vi "Break on Unsupported Target.vi"   [LabVIEW 2020, in "common.lvlib"]
uses:
  common.lvlib
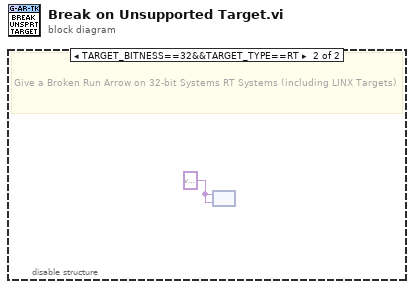
[diagram p0: block diagram]
diagram:
  n1 = disable-structure shown="TARGET_BITNESS==32&&TARGET_TYPE==RT" {
    frame condition #0 (active) {
      # "Not 32-Bit - All Good"
    }
    frame condition #1 {
      w1 = variant ("type")
      # "Give a Broken Run Arrow on 32-bit Systems RT Systems (including LINX Targets)"
      n2 = node(w1, w1) -> ()  [unwired: 1 out]
    }
  }
